vi "Destroy.vi"(0 "reference":refnum<class "ActorNode.lvclass">, 5 "error in (no error)":errorcluster) -> (15 "# of objects":i32, 19 "error out":errorcluster)   [LabVIEW 2012, in "ActorNode.lvclass"]
doc: "Destroys a ActorNode object created with a ActorNode constructor VI.\n\n[GOOP 2.1]"
uses:
  <resource>/Framework/Providers/Open_GDS/UML/ActorNode_class/ActorNode.lvclass
  <resource>/Framework/Providers/Open_GDS/UML/RectangularNode_class/RectangularNode.lvclass
  <resource>/Framework/Providers/Open_GDS/UML/MultiLineString_class/MultiLineString.lvclass
panel:
  out "reference out":refnum<class "ActorNode.lvclass">
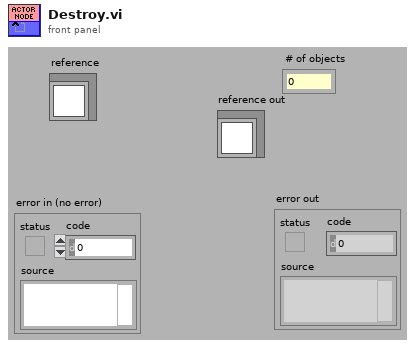
[diagram p1: front panel]
types:
  T1 = typedef "ActorNode.lvclass/ObjectAttributes.ctl" = cluster{"Base class":T2, "name":refnum<class "MultiLineString.lvclass">, "DEFAULT_WIDTH":i32, "DEFAULT_HEIGHT":i32, "DEFAULT_GAP":i32}
  T2 = typedef "RectangularNode.lvclass/ObjectAttributes.ctl" = cluster{"Base class":T3, "bounds":T4}
  T3 = typedef "AbstractNode.lvclass/ObjectAttributes.ctl" = cluster{"parent":refnum<class "AbstractNode.lvclass">, "children":refnum<class "AbstractNode.lvclass">[], "Hidden":bool}
  T4 = typedef "Rectangle Rectangle2D.ctl" = cluster{"x":dbl, "y":dbl, "width":dbl, "height":dbl}
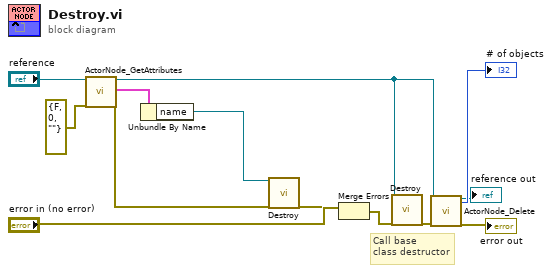
[diagram p0: block diagram]
diagram:
  # "Call base\nclass destructor"
  n1 = call <resource>:"ActorNode_GetAttributes.vi"("reference in"="reference", "error in (no error)"=errorcluster {"status"=FALSE, "code"=0, "source"=""}) -> ("reference out"=w2:refnum<class "ActorNode.lvclass">, "Attributes"=w8:T1, "error out"=w5:errorcluster)  [unwired: 15 out]
  n2 = Unbundle By Name(w8) -> ("name"=w7:refnum<class "MultiLineString.lvclass">)
  n3 = call-dynamic "Destroy.vi"("reference"=w7, "error in (no error)"=w5) -> ("error out"=w6:errorcluster)  [unwired: 16 in, 1 out]
  n4 = Merge Errors("error in (no error)", w6) -> (w3:errorcluster)
  n5 = call-parent "Destroy.vi"("reference"=w2, "error in (no error)"=w3) -> ("error out"=w1:errorcluster)  [unwired: 16 in, 1 out]
  n6 = call <resource>:"ActorNode_Delete.vi"("reference in"=w2, "error in (no error)"=w1) -> ("reference out"=→"reference out":refnum<class "ActorNode.lvclass">, "# of objects"=→"# of objects":i32, "error out"=→"error out":errorcluster)  [unwired: 15 out]
